vi "4-1.vi"() -> ()   [LabVIEW 2014]
panel:
  out "error out":errorcluster
  in  "error in (no error)":errorcluster
  in  "Current Temp":dbl
  in  "Min Temp":dbl
  in  "Max Temp":dbl
  out "Warning?":bool
  out "Warning Text":string
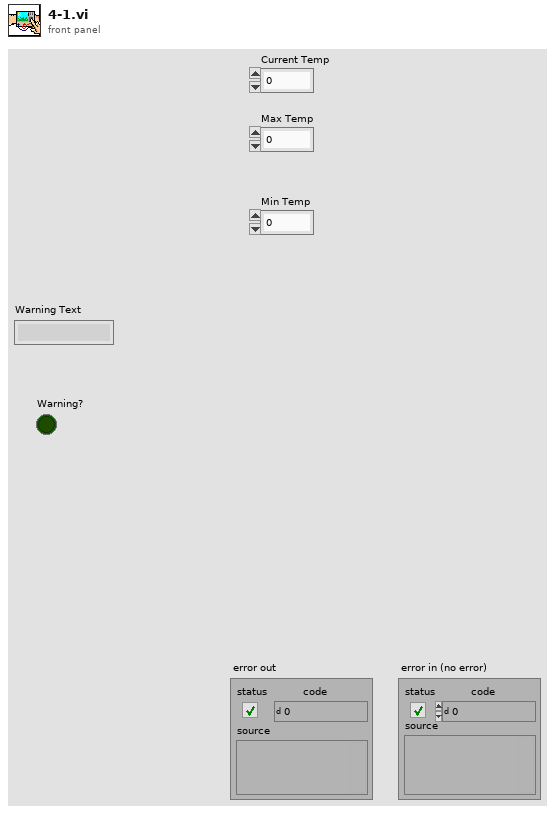
[diagram p1: front panel]
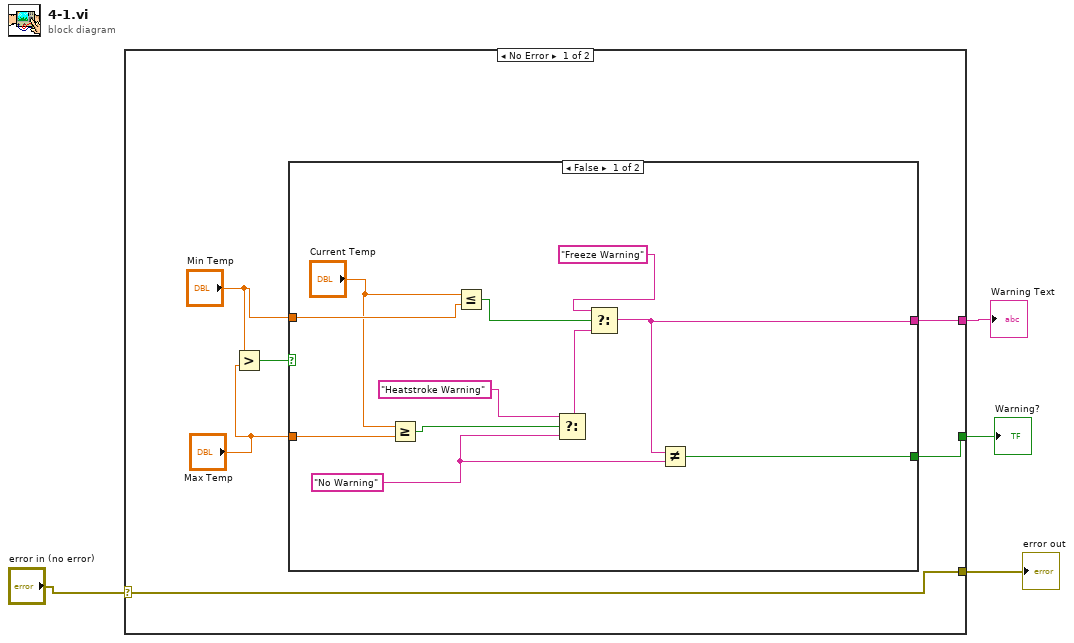
[diagram p0: block diagram]
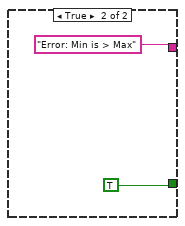
[diagram p2: hidden frame]
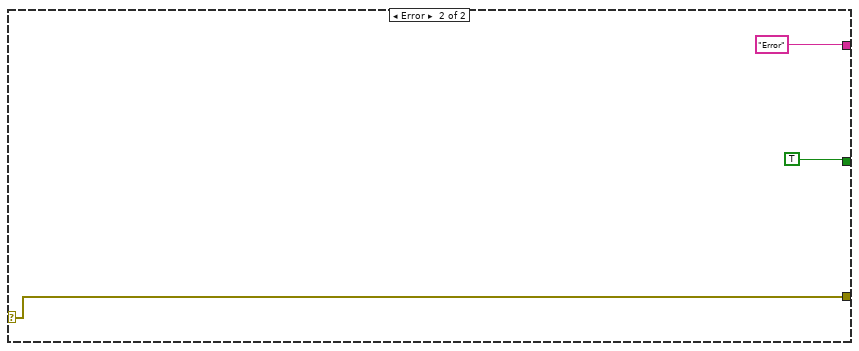
[diagram p3: hidden frame]
diagram:
  n1 = case shown="No Error" "error in (no error)" {
    selector: "error in (no error)" -> [w5 w26]
    tunnel: [w7 "Error"] -> w4
    tunnel: [w6 TRUE] -> w3
    tunnel: [w5 w26] -> w1
    frame No Error {
      n2 = Greater?(x="Min Temp", y="Max Temp") -> (0:w8:bool)
      n3 = case shown="False" w8 {
        tunnel: "Min Temp" -> [w15 _]
        tunnel: "Max Temp" -> [w14 _]
        tunnel: [w12 TRUE] -> w6
        tunnel: [w11 "Error: Min is > Max"] -> w7
        frame False {
          w18 = "No Warning"
          n4 = Greater Or Equal?(x="Current Temp", y=w14) -> (x >= y?=w19:bool)
          n5 = Less Or Equal?(x="Current Temp", y=w15) -> (x <= y?=w16:bool)
          n6 = Select(t="Heatstroke Warning", s=w19, f=w18) -> (s? t:f=w17:string)
          n7 = Select(t="Freeze Warning", s=w16, f=w17) -> (s? t:f=w11:string)
          n8 = Not Equal?(x=w11, y=w18) -> (x != y?=w12:bool)
        }
        frame True {
        }
      }
    }
    frame Error {
    }
  }
  "Warning?" <- w3
  "Warning Text" <- w4
  "error out" <- w1
